vi "calcEffGQFWHM.vi"(8 "error in (no error)":errorcluster, 9 "Field Idx":i32[](array[numeric]), 10 "PSSN":dbl[](array[numeric]), 11 "OptCtrl in":refnum<class "OptCtrl.lvclass">) -> (0 "error out":errorcluster, 2 "Effective GQFWHM (arcsec)":dbl, 3 "OptCtrl out":refnum<class "OptCtrl.lvclass">)   [LabVIEW 2016, in "OfcFunc.lvlib" / "OptCtrl.lvclass"]
doc: "Calculate the effective full width at halh maximum (FWHM) by Gaussian quadrature."
uses:
  OptCtrl.lvclass
  MatOper/getSubArray1D.vi
  MatOper/MatOper.lvclass
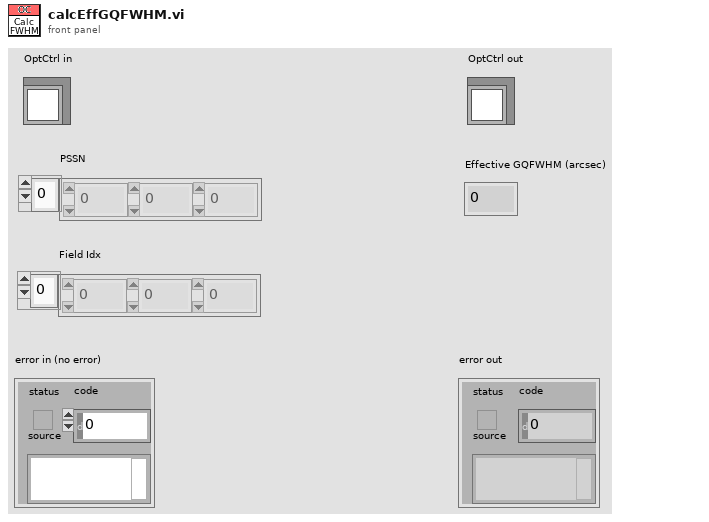
[diagram p1: front panel]
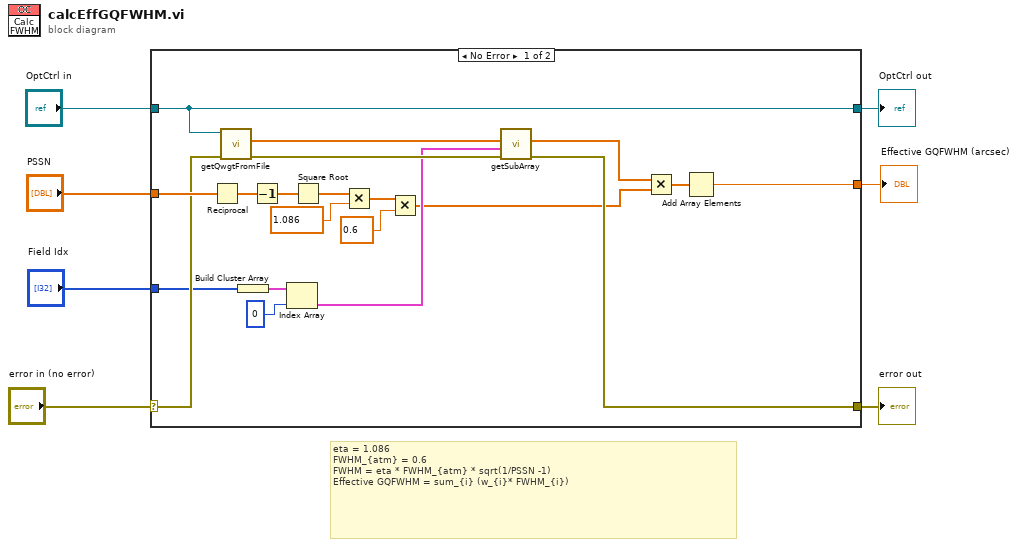
[diagram p0: block diagram]
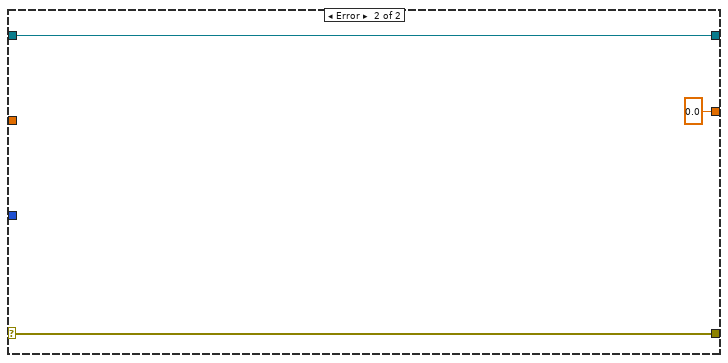
[diagram p2: hidden frame]
diagram:
  # "eta = 1.086\nFWHM_{atm} = 0.6\nFWHM = eta * FWHM_{atm} * sqrt(1/PSSN -1)\nEffective GQFWHM = sum_{i} (w_{i}* FWHM_{i})"
  n1 = case shown="No Error" "error in (no error)" {
    selector: "error in (no error)" -> [w20 w30]
    tunnel: [w16 w30] -> w6
    tunnel: [w19 w29] -> w4
    tunnel: "OptCtrl in" -> [w19 w29]
    tunnel: "PSSN" -> [w27 _]
    tunnel: "Field Idx" -> [w13 _]
    tunnel: [w8 0.0] -> w1
    frame No Error {
      n2 = Reciprocal(x=w27) -> (1/x=w26:dbl[])
      n3 = call "getQwgtFromFile.vi"("error in (no error)"=w20, "OptCtrl in"=w19) -> ("error out"=w17:errorcluster, "Wgt of Q"=w18:dbl[])  [unwired: 7 in, 1 out]
      n4 = Build Cluster Array(w13) -> (w15:cluster{"Field Idx":i32[]}[])
      n5 = Decrement(x=w26) -> (x-1=w25:dbl[])
      n6 = Index Array(array=w15, index=0) -> (element=w12:cluster{"Field Idx":i32[]})
      n7 = Square Root(x=w25) -> (sqrt(x)=w24:dbl[])
      n8 = Multiply(x=w24, y=1.086) -> (x*y=w23:dbl[])
      n9 = Multiply(x=w23, y=0.6) -> (x*y=w10:dbl[])
      n10 = call-poly "getSubArray.vi"("error in (no error)"=w17, "Index Array Cluster"=w12, "1D Array"=w18) -> ("error out"=w16:errorcluster, "Sub-Array"=w11:dbl[])  [unwired: 6 in, 1 out]
      n11 = Multiply(x=w11, y=w10) -> (x*y=w9:dbl[])
      n12 = Add Array Elements(numeric array=w9) -> (sum=w8:dbl)
    }
    frame Error {
    }
  }
  "error out" <- w6
  "OptCtrl out" <- w4
  "Effective GQFWHM (arcsec)" <- w1
